vi "Resize Diagram Window.vi"(6 "Variant in":variant, 7 "Shift Pressed?":bool, 8 "error in (no error)":errorcluster, 10 "QD Combo Box Ref":refnum<vi>, 11 "QD Launch VI Ref":refnum<vi>) -> (0 "error out":errorcluster, 4 "Variant out":variant)   [LabVIEW 2019]
doc: "Resize the block diagram to content.\n\nCreated by: Ryan Pacini\n\nDefault Shortcut - [E]"
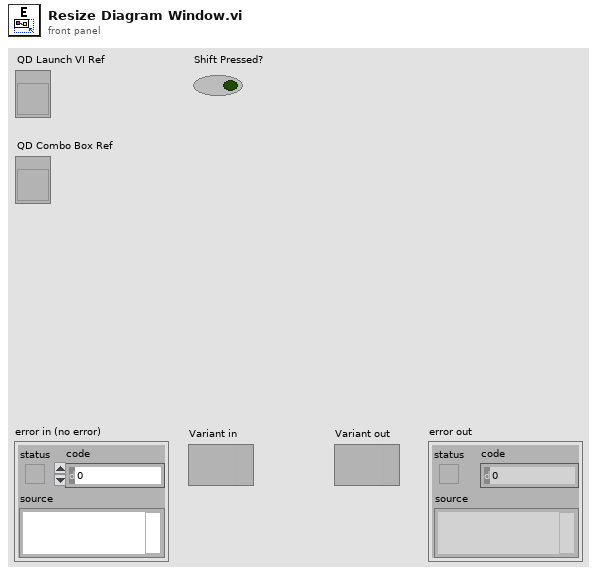
[diagram p1: front panel]
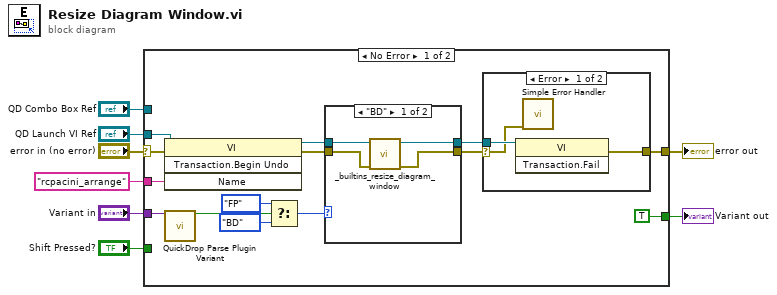
[diagram p0: block diagram]
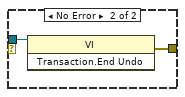
[diagram p3: hidden frame]
diagram:
  n1 = case shown="No Error" "error in (no error)" {
    selector: "error in (no error)" -> [w22 w34]
    tunnel: [w21 w34] -> w3
    tunnel: "QD Launch VI Ref" -> [w17 _]
    tunnel: "rcpacini_arrange" ("Undo Name") -> [w20 _]
    tunnel: "Variant in" -> [w18 _]
    tunnel: [TRUE _] -> w4
    tunnel: "QD Combo Box Ref" -> [_ _]
    tunnel: "Shift Pressed?" -> [_ _]
    frame No Error {
      n2 = invoke class="VI" method="Transaction.Begin Undo"(reference=w17, error in=w22, "Name"=w20) -> (reference out=w16:refnum<vi>, error out=w15:errorcluster)  [unwired: 1 in, 2 out]
      n3 = call <vilib>:"QuickDrop Parse Plugin Variant.vi"("QDKS Variant in"=w18) -> ("QD Launch VI Panel?"=w12:bool)  [unwired: 12 in, 2 out]
      n4 = Select(t=enum8{"FP", "BD"}."FP" ("Panel"), s=w12, f=enum8{"FP", "BD"}."BD" ("Panel")) -> (s? t:f=w10:enum8{"FP", "BD"})
      n5 = case shown="\"BD\"" w10 {
        tunnel: w16 -> [w26 w28]
        tunnel: w15 -> [w24 w27]
        tunnel: [w25 w28] -> w11
        tunnel: [w23 w27] -> w9
        frame "BD" {
          n6 = call "_builtins_resize_diagram_window.vi"("error in (no error)"=w24, "VI Refnum in"=w26) -> ("error out"=w23:errorcluster, "VI Refnum out"=w25:refnum<vi>)  [unwired: 8 in]
        }
        frame "FP" {
        }
      }
      n7 = case shown="Error" w9 {
        selector: w9 -> [w29 _]
        tunnel: w11 -> [w30 w32]
        tunnel: [w31 w33] -> w21
        frame Error {
          n8 = invoke class="VI" method="Transaction.Fail"(reference=w30) -> (error out=w31:errorcluster)  [unwired: 2 in, 2 out]
          n9 = call <vilib>:"Simple Error Handler.vi"("error in (no error)"=w29) -> ()  [unwired: 4 in, 5 out]
        }
        frame No Error {
          n10 = invoke class="VI" method="Transaction.End Undo"(reference=w32) -> (error out=w33:errorcluster)  [unwired: 2 in, 2 out]
        }
      }
    }
    frame Error {
    }
  }
  "error out" <- w3
  "Variant out" <- w4
